vi "Strassen_Punkte.vi"(10 "Strassen":T1[](array[typedef]), 11 "Kreuzungen":T4[](array[typedef])) -> (3 "Strassenpunkte":T6[](array[typedef]))   [LabVIEW 2019]
uses:
  2_Pt_Strasse.ctl
  Koordinate.ctl
  Kreuzung.ctl
  Strasse.ctl
  Verbindung.ctl
  Strassentyp.ctl
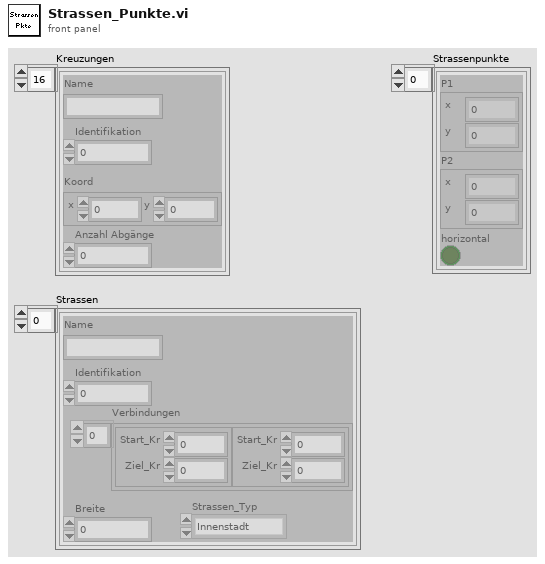
[diagram p1: front panel]
types:
  T1 = typedef "Strasse.ctl" = cluster{"Name":string, "Identifikation":u8, "Verbindungen":T2[], "Breite":u8, "Strassen_Typ":T3}
  T2 = typedef "Verbindung.ctl" = cluster{"Start_Kr":u16, "Ziel_Kr":u16}
  T3 = typedef "Strassentyp.ctl" = enum16{"Innenstadt", "Stadt", "Land"}
  T4 = typedef "Kreuzung.ctl" = cluster{"Name":string, "Identifikation":u8, "Koord":T5, "Anzahl Abgänge":u8}
  T5 = typedef "Koordinate.ctl" = cluster{"x":dbl, "y":dbl}
  T6 = typedef "2_Pt_Strasse.ctl" = cluster{"P1":T5, "P2":T5, "horizontal":bool}
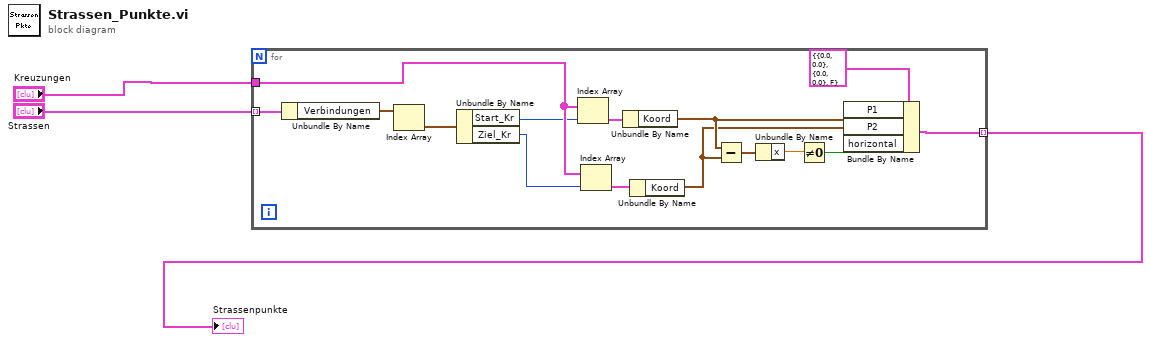
[diagram p0: block diagram]
diagram:
  n1 = for {
    tunnel: "Strassen" -> [w18] mode=indexing
    tunnel: "Kreuzungen" -> [w15]
    tunnel: [w5] -> w3 mode=indexing
    n2 = Unbundle By Name(w18) -> ("Verbindungen"=w17:T2[])
    n3 = Index Array(array=w17) -> (element=w16:T2)  [unwired: 1 in]
    n4 = Unbundle By Name(w16) -> ("Start_Kr"=w14:u16, "Ziel_Kr"=w13:u16)
    n5 = Index Array(array=w15, index=w14) -> (element=w12:T4)
    n6 = Index Array(array=w15, index=w13) -> (element=w11:T4)
    n7 = Unbundle By Name(w12) -> ("Koord"=w8:T5)
    n8 = Unbundle By Name(w11) -> ("Koord"=w7:T5)
    n9 = Subtract(x=w8, y=w7) -> (x-y=w10:T5)
    n10 = Unbundle By Name(w10) -> ("x"=w9:dbl)
    n11 = Not Equal To 0?(x=w9) -> (x != 0?=w6:bool)
    n12 = Bundle By Name(cluster=T6 {"P1"={"x"=0.0, "y"=0.0}, "P2"={"x"=0.0, "y"=0.0}, "horizontal"=FALSE} ("strasse"), "P1"=w8, "P2"=w7, "horizontal"=w6) -> (w5:T6)
  }
  "Strassenpunkte" <- w3
